vi "Actor Core.vi"(8 "error in":errorcluster, 11 "tWorkerTCPConnection in":refnum<class "tWorkerTCPConnection.lvclass">) -> (0 "error out":errorcluster, 3 "Actor out":refnum<class "Actor.lvclass">)   [LabVIEW 2013, in "tWorkerTCPConnection.lvlib" / "tWorkerTCPConnection.lvclass"]
doc: "(<B>Filename</B>: Actor Framework.lvlib:Actor.lvclass:Actor Core.vi)\n\nReceives messages to the actor, reacts to them, and initiates any error handling that may shut the actor down.\n\nDescendant classes may override this VI to append parallel tasks for the actor to complete while it handles messages. Overrides use the Call Parent Method node."
uses:
  tWorkerTCPConnection.lvclass
  <vilib>/ActorFramework/Actor/Actor.lvclass
  tWorkerCommandRunner/tWorkerCommandRunner/tWorkerCommandRunner.lvclass
  <vilib>/ActorFramework/Actor/Actor.lvclass/Actor.ctl
  <vilib>/ActorFramework/Message Enqueuer/Message Enqueuer.lvclass/Message Enqueuer.ctl
  tWorkerTCPConnection.lvclass/tWorkerTCPConnection.ctl
  msgs/Process Message Msg/Process Message Msg.lvclass/Process Message Msg.ctl
  <vilib>/ActorFramework/Message Enqueuer/Init from Existing Queue.vi
  <vilib>/ActorFramework/Message Enqueuer/Enqueue.vi
  <vilib>/ActorFramework/Message Priority Queue/Priority Enqueue.vi
  <vilib>/ActorFramework/Message Enqueuer/Message Enqueuer.lvclass
  msgs/Process Message Msg/Process Message Msg.lvclass
  <vilib>/ActorFramework/Stop Msg/Stop Msg.lvclass
  BSON/BSON.lvlib
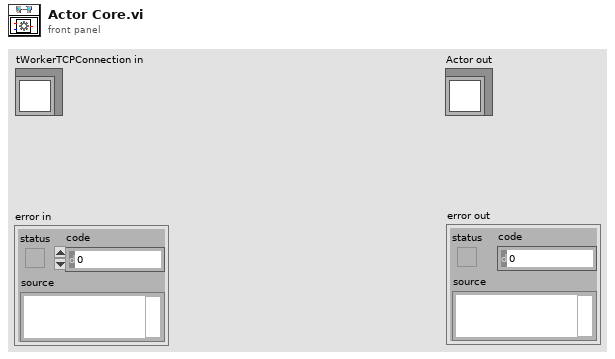
[diagram p1: front panel]
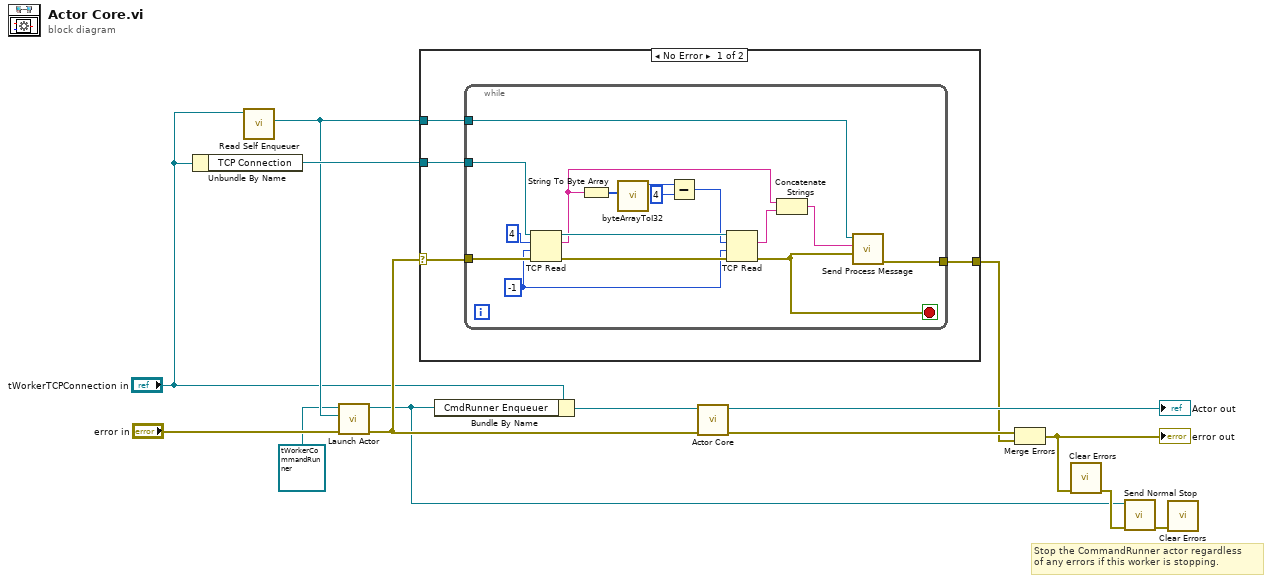
[diagram p0: block diagram]
diagram:
  # "Stop the CommandRunner actor regardless\nof any errors if this worker is stopping."
  n1 = Unbundle By Name("tWorkerTCPConnection in") -> ("TCP Connection"=w13:refnum<k5>)
  n2 = call <vilib>:"Read Self Enqueuer.vi"("Actor"="tWorkerTCPConnection in") -> ("Self Enqueuer"=w9:refnum<class "Message Enqueuer.lvclass">)  [unwired: 10 in]
  n3 = call <vilib>:"Launch Actor.vi"("error in (no error)"="error in", "Actor-to-Caller Enqueuer"=w9, "Actor"=refnum<class "tWorkerCommandRunner.lvclass"> refnum ("tWorkerCommandRunner.lvlib:tWorkerCommandRunner.lvclass")) -> ("error out"=w7:errorcluster, "Caller-To-Actor Enqueuer"=w2:refnum<class "Message Enqueuer.lvclass">)  [unwired: 7 in]
  n4 = case shown="No Error" w7 {
    selector: w7 -> [w17 _]
    tunnel: w13 -> [w18 _]
    tunnel: w9 -> [w16 _]
    tunnel: [w15 _] -> w11
    frame No Error {
      n5 = while {
        tunnel: w18 -> [w26]
        tunnel: w17 -> [w25]
        tunnel: w16 -> [w22]
        tunnel: [w19] -> w15
        stop <- w20 stop-if-true
        w23 = -1 ("timeout ms (25000)")
        n6 = TCP Read(connection ID=w26, bytes to read=4, error in (no error)=w25, 9:w23) -> (connection ID out=w30:refnum<k5>, data out=w28:string, error out=w24:errorcluster)  [unwired: 1 in]
        n7 = String To Byte Array(string=w28) -> (unsigned byte array=w31:u8[])
        n8 = call "byteArrayToI32.vi"("ByteArrayIn"=w31) -> ("I32"=w32:i32)  [unwired: 7 in, 3 out]
        n9 = Subtract(x=w32, y=4) -> (x-y=w29:i32)
        n10 = TCP Read(connection ID=w30, bytes to read=w29, error in (no error)=w24, 9:w23) -> (data out=w27:string, error out=w20:errorcluster)  [unwired: 1 in, 1 out]
        n11 = Concatenate Strings(w28, w27) -> (w21:string)
        n12 = call "Send Process Message.vi"("Error From Read"=w20, "Message"=w21, "Message Enqueuer"=w22) -> ("error out"=w19:errorcluster)  [unwired: 7 in, 1 out]
      }
    }
    frame Error {
    }
  }
  n13 = Bundle By Name(cluster="tWorkerTCPConnection in", "CmdRunner Enqueuer"=w2) -> (w5:refnum<class "tWorkerTCPConnection.lvclass">)
  n14 = call-parent "Actor Core.vi"("error in"=w7, "Actor in"=w5) -> ("error out"=w12:errorcluster, "Actor out"=→"Actor out":refnum<class "Actor.lvclass">)  [unwired: 8 in]
  n15 = Merge Errors(w12, w11) -> (w4:errorcluster)
  "error out" <- w4
  n16 = call <vilib>:"Clear Errors.vi"("error in (no error)"=w4) -> ("error out"=w3:errorcluster)  [unwired: 6 in]
  n17 = call <vilib>:"Send Normal Stop.vi"("error in (no error)"=w3, "Message Enqueuer"=w2) -> ("error out"=w1:errorcluster)  [unwired: 9 in]
  n18 = call <vilib>:"Clear Errors.vi"("error in (no error)"=w1) -> ()  [unwired: 6 in, 1 out]
